vi "Save Hologram As Dbl v2.vi"   [LabVIEW 2014]
types:
  T1 = cluster{"[0]":i32, "[1]":i32, "[2]":i32, "[3]":i32}
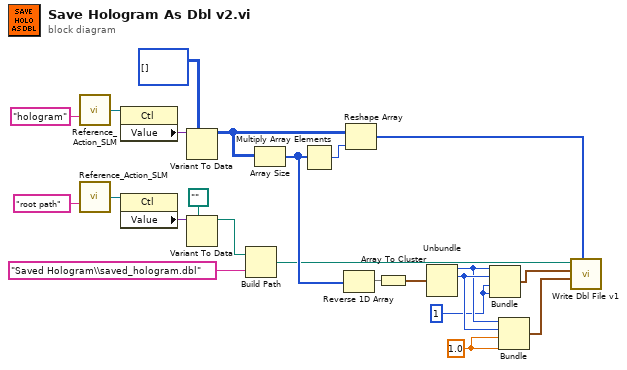
[diagram p0: block diagram]
diagram:
  w14 = 1
  w11 = 1.0
  n1 = call "Reference_Action_SLM.vi"("Control Name"="hologram") -> ("Ref OUT"=w22:refnum<vi>)  [unwired: 12 in, 2 out]
  n2 = call "Reference_Action_SLM.vi"("Control Name"="root path") -> ("Ref OUT"=w7:refnum<vi>)  [unwired: 12 in, 2 out]
  n3 = property class="Ctl"(reference=w22) -> ("Value"=w21:variant)  [unwired: 1 in, 2 out]
  n4 = property class="Ctl"(reference=w7) -> ("Value"=w6:variant)  [unwired: 1 in, 2 out]
  n5 = Variant To Data(type=u8[][] [], Variant=w21) -> (data=w18:u8[][])  [unwired: 1 in, 1 out]
  n6 = Variant To Data(type=path "" ("appended path"), Variant=w6) -> (data=w4:path)  [unwired: 1 in, 1 out]
  n7 = Build Path(base path=w4, name or relative path="Saved Hologram\\saved_hologram.dbl" ("string")) -> (appended path=w2:path)
  n8 = Array Size(array=w18) -> (size(s)=w9:i32[])
  n9 = Multiply Array Elements(1:w9) -> (0:w19:i32)
  n10 = Reverse 1D Array(array=w9) -> (reversed array=w10:i32[])
  n11 = Reshape Array(w18, w19) -> (w1:u8[])
  n12 = Array To Cluster(array=w10) -> (cluster=w13:T1)
  n13 = Unbundle(w13) -> ("[0]"=w16:i32, "[1]"=w17:i32)  [unwired: 2 out]
  n14 = Bundle("[0]"=w16, "[1]"=w17, w14, w14) -> (w15:cluster{"[0]":i32, "[1]":i32, i32, i32})  [unwired: 1 out]
  n15 = Bundle("[0]"=w16, "[1]"=w17, w11, w11) -> (w12:cluster{"[0]":i32, "[1]":i32, dbl, dbl})  [unwired: 1 out]
  n16 = call "Write Dbl File v1.vi"("data"=w1, "axis lengths"=w12, "pixel numbers"=w15, "Path"=w2) -> ()  [unwired: 5 in, 1 out]
